vi "Step(Tape).vi"(8 "error in (no error)":errorcluster, 11 "TapeDrive in":refnum<class "TapeDrive.lvclass">) -> (0 "error out":errorcluster, 1 "trajectories":dbl[][](graph)=[[1.0, 0.7046880791959296, 0.4965852858533471, 0.3499377259476329, 0.2465969370957652, 0.1737739140097176, 0.12245639698366893, 0.08629355394147512, 0.06081002915927391, 0.0628100291592739, 0.0648100291592739, 0.0668100291592739, 0.06881002915927391, 0.08881002915927391, 0.12881002915927392, 0.18881002915927392, 0.26881002915927393, 0.36881002915927397, 0.48881002915927396, 0.628810029159274, 0.788810029159274, 0.968810029159274, 1.0], [0.0, 0.0, 0.0, 0.0, 0.0, 0.0, 0.004000000000814907, 0.002999999998792191, 0.040000000000873115, 0.20499999999992724, 0.363999999999578, 0.5879999999997381, 0.7160000000003492, 0.7360000000007858, 0.7879999999986467, 0.6760000000012951, 0.3989999999994325, 0.01300000000082946, 0.004000000000814907, 0.003999999998995918, 0.0, 0.0, 0.0], [0.0, 0.0, 0.0, 0.0, 0.0, 0.0, 0.004000000000814907, -0.0010000000020227162, 0.037000000002080924, 0.16499999999905413, 0.15899999999965075, 0.22400000000016007, 0.12800000000061118, 0.020000000000436557, 0.05199999999786087, -0.11199999999735155, -0.27700000000186265, -0.385999999998603, -0.009000000000014552, -1.8189894035458565e-12, -0.003999999998995918, 0.0, 0.0]], 3 "TapeDrive out":refnum<class "TapeDrive.lvclass">, 4 "ok":bool, 5 "position":dbl)   [LabVIEW 2020, in "TapeDrive.lvclass"]
uses:
  TapeDrive.lvclass
  TapeDrive.lvclass/TapeDrive.ctl
  Newport ESP301.lvlib
panel:
  out "maxVel":dbl[](graph)
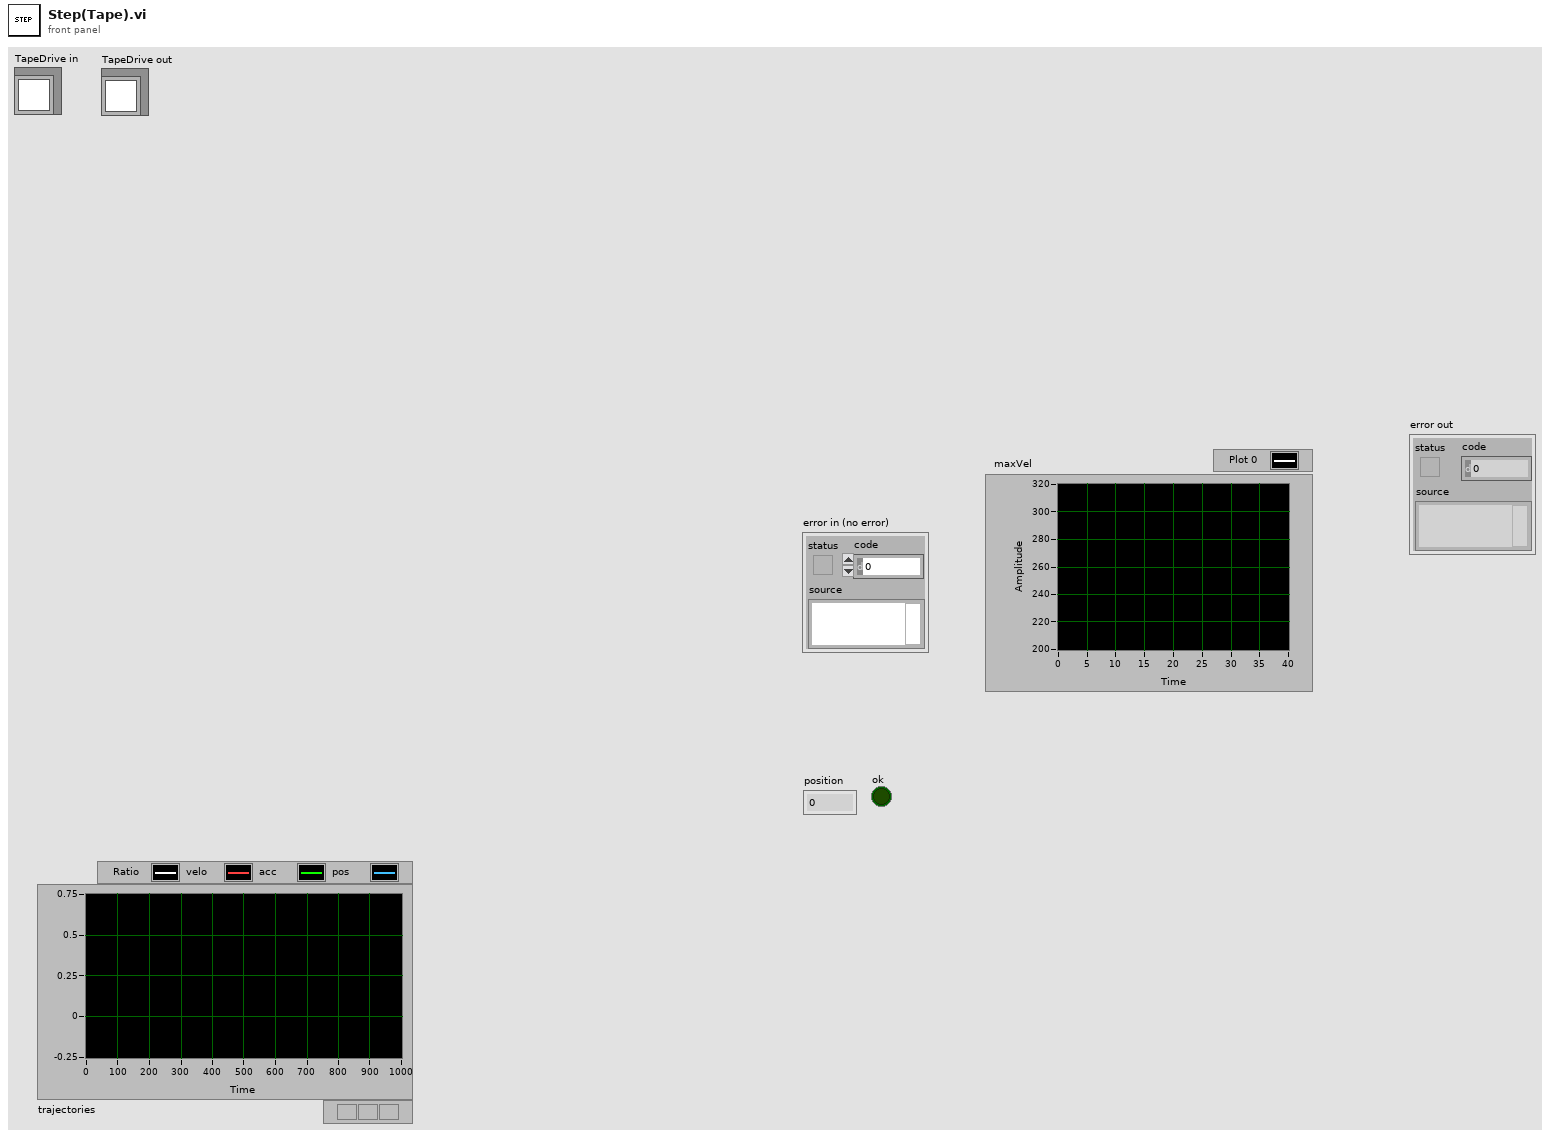
[diagram p1: front panel]
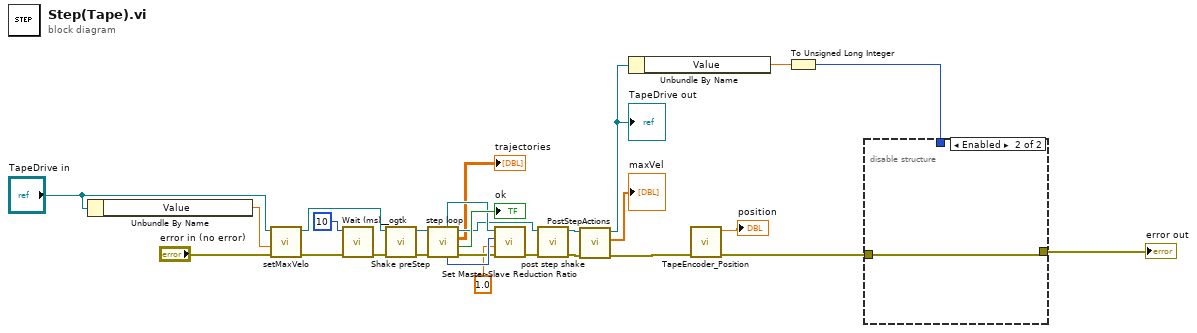
[diagram p0: block diagram]
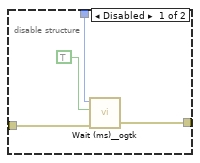
[diagram p2: hidden frame]
diagram:
  n1 = Unbundle By Name("TapeDrive in") -> ("Value"=w14:dbl)
  n2 = call "setMaxVelo.vi"("error in (no error)"="error in (no error)", "NewVal"=w14, "TapeDrive in"="TapeDrive in") -> ("error out"=w16:errorcluster, "TapeDrive out"=w11:refnum<class "TapeDrive.lvclass">)  [unwired: 6 in, 1 out]
  n3 = call "Wait (ms)__ogtk.vi"("error in (no error)"=w16, "milliseconds to wait"=u32 10) -> ("error out"=w1:errorcluster)  [unwired: 8 in, 1 out]
  n4 = call "Shake preStep.vi"("error in (no error)"=w1, "TapeDrive in"=w11) -> ("error out"=w17:errorcluster, "TapeDrive out"=w6:refnum<class "TapeDrive.lvclass">)  [unwired: 8 in]
  n5 = call "step loop.vi"("error in (no error)"=w17, "TapeDrive in"=w6) -> ("error out"=w19:errorcluster, "Boolean"=→"ok":bool, "trajectories"=→"trajectories":dbl[][], "TapeDrive out"=w10:refnum<class "TapeDrive.lvclass">, "Slave"=w20:i32, "VISA Refnum out"=w21:refnum<visa-resource-name>)  [unwired: 4 in]
  n6 = call "Set Master-Slave Reduction Ratio.vi"("error in (no error)"=w19, "Reduction Ratio (0)"=1.0, "Axis (1)"=w20, "VISA resource name"=w21) -> ("error out"=w18:errorcluster)  [unwired: 2 in, 1 out]
  n7 = call "post step shake.vi"("error in (no error)"=w18, "TapeDrive in"=w10) -> ("error out"=w8:errorcluster, "TapeDrive out"=w9:refnum<class "TapeDrive.lvclass">)  [unwired: 8 in]
  n8 = call "PostStepActions.vi"("error in (no error)"=w8, "TapeDrive in"=w9) -> ("error out"=w7:errorcluster, "maxVel"=→"maxVel":dbl[], "TapeDrive out"=w4:refnum<class "TapeDrive.lvclass">)  [unwired: 7 in]
  "TapeDrive out" <- w4
  n9 = Unbundle By Name(w4) -> ("Value"=w3:dbl)
  n10 = call "TapeEncoder_Position.vi"("error in (no error)"=w7) -> ("error IO"=w24:errorcluster, "position"=→"position":dbl)  [unwired: 9 in]
  n11 = To Unsigned Long Integer(number=w3) -> (unsigned 32bit integer=w22:u32)
  n12 = disable-structure shown="Enabled" {
    disable-tunnel: [w31 w32] -> w26
    disable-tunnel: w24 -> [w30 w32]
    disable-tunnel: w22 -> [w28 _]
    frame Disabled {
      n13 = call "Wait (ms)__ogtk.vi"("error in (no error)"=w30, "Wait on Error (FALSE)"=TRUE, "milliseconds to wait"=w28) -> ("error out"=w31:errorcluster)  [unwired: 7 in, 1 out]
    }
    frame Enabled {
    }
  }
  "error out" <- w26
